vi "Log name String to Display.vi"(11 "Log Name":string) -> (2 "Date":string, 3 "Day":string)   [LabVIEW 2019]
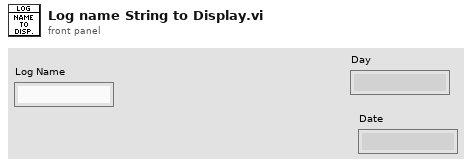
[diagram p1: front panel]
types:
  T1 = typedef "LVDateTimeRec.ctl" = cluster{"fractional second":dbl, "second":i32, "minute":i32, "hour":i32, "day of month":i32, "month":i32, "year":i32, "day of week":i32, "day of year":i32, "DST":i32}
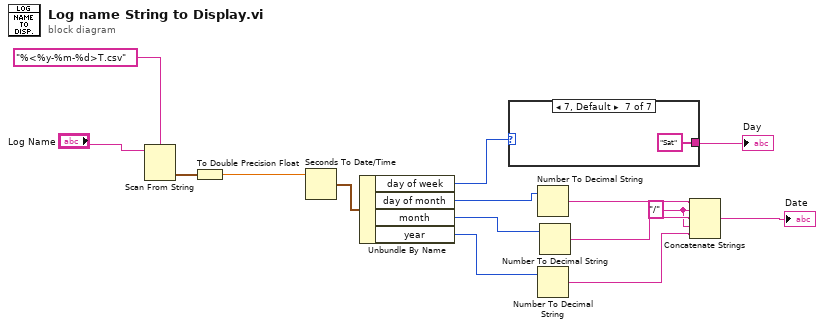
[diagram p0: block diagram]
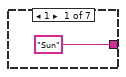
[diagram p2: hidden frame]
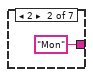
[diagram p3: hidden frame]
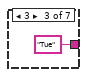
[diagram p4: hidden frame]
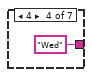
[diagram p5: hidden frame]
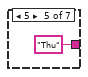
[diagram p6: hidden frame]
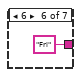
[diagram p7: hidden frame]
diagram:
  w3 = "/" ("element")
  n1 = Scan From String(format string="%<%y-%m-%d>T.csv", input string="Log Name") -> (output 1=w13:timestamp)  [unwired: 3 in, 3 out]
  n2 = To Double Precision Float(number=w13) -> (double precision float=w12:dbl)
  n3 = Seconds To Date/Time(time stamp (now)=w12) -> (date time rec=w11:T1)  [unwired: 1 in]
  n4 = Unbundle By Name(w11) -> ("day of week"=w10:i32, "day of month"=w8:i32, "month"=w7:i32, "year"=w6:i32)
  n5 = case shown="7, Default" w10 {
    tunnel: ["Sun" "Mon" "Tue" "Wed" "Thu" "Fri" "Sat"] -> w9
    frame 1 {
    }
    frame 2 {
    }
    frame 3 {
    }
    frame 4 {
    }
    frame 5 {
    }
    frame 6 {
    }
    frame 7, Default {
    }
  }
  "Day" <- w9
  n6 = Number To Decimal String(number=w8) -> (decimal integer string=w5:string)  [unwired: 1 in]
  n7 = Number To Decimal String(number=w6) -> (decimal integer string=w2:string)  [unwired: 1 in]
  n8 = Number To Decimal String(number=w7) -> (decimal integer string=w4:string)  [unwired: 1 in]
  n9 = Concatenate Strings(w5, w3, w4, w3, w2) -> (→"Date":string)
